vi "FPGA myRIOMain_v7.vi"() -> ()   [LabVIEW 2019]
doc: "Main FPGA VI\nUse the bitfile generated by this VI in the real-time code.\n\nv5: 16-pt Moving Average filter in AI sample loop"
uses:
  <vilib>/eio/EIONode/EIONode.xnode
  <vilib>/rvi/DataTransferAndStorage/Container/XNode/niFpgaContainer.xnode
  <vilib>/rvi/eio/common/nirviEmuTemplateMethod_errors.vi
  <vilib>/rvi/FIFO/Fifo_Resource/nirvififoEmulationRead.vi
  <vilib>/rvi/FIFO/Fifo_Resource/nirvififoEmulationWrite.vi
  FPGA functions/FPGA functions.lvlib
  <vilib>/rvi/FXPMathLib/FxpMul/XNode/nifxpmath_Multiplier.xnode
  <vilib>/rvi/DataTransferAndStorage/Register/Emulation/niFpgaRegisterEmulation.vi
  <vilib>/rvi/Analysis/measure/LMRsmpl/XNode/niFPGA Rational Resampler.xnode
  <vilib>/Platform/TimedLoop/XDataNode/wakeup.ctl
  <vilib>/Platform/TimedLoop/XDataNode/XDNodeRunTimeDep.lvlib
  <vilib>/Platform/TimedLoop/XDataNode/nitl_modes.ctl
  <vilib>/Platform/TimedLoop/XDataNode/timing_clust.ctl
  <vilib>/Platform/TimedLoop/XDataNode/XDataNode.xnode
  <vilib>/rvi/Analysis/common/codeGenErrors/XNode/niFpgaXNodeCodeGenErrorHandle.vi
  <vilib>/rvi/FXPMathLib/sim/FxpSim.dll
  TypeDefs/AO mode TabCtrl.ctl
  TypeDefs/SamplingModeEnum.ctl
panel:
  out "FPGA Proc. \nDMA\nOverflow?":bool
  out "AI M Loop time [ticks]":u32
  out "FPGA AI DMA\nOverflow?":bool
  out "Sample Freq. \ntoo high?":bool
  out "Processing Loop time [ticks]":u32
  in  "Sampling Mode":T1
  in  "AO mode":T2
  in  "AO Out [V]":fxp<+/-,18,5> format="%#.6g"
  in  "AO enable?":bool
  out "AI In [V]":fxp<+/-,24,5> format="%#.6g"
  out "FPGA AO DMA\nOverflow?":bool
  out "Int. Output":i16
  out "Raw Int. Input":fxp<+/-,20,12> format="%.8g"
  out "AO Loop time [ticks]":u32
  out "AI Loop time [ticks]":u32
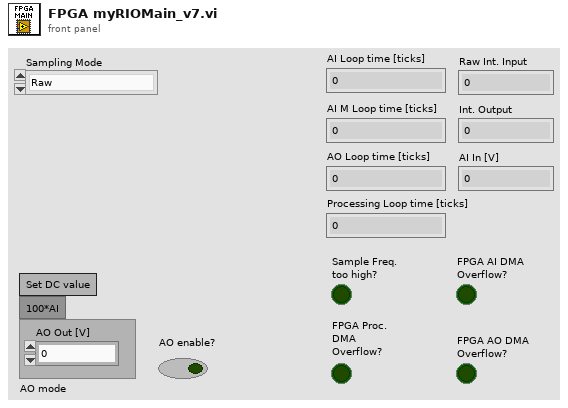
[diagram p1: front panel]
types:
  T1 = typedef "SamplingModeEnum.ctl" = enum16{"Raw", "M64 (ReSpl)", "M128 (ReSpl)", "M256 (ReSpl)", "MA (AI)", "4pt MA (AI) + M64 (ReSpl)", "LPF (Proc.)", "4pt MA (AI) + LPF (Proc.)", "4pt MA (Proc.) + LPF (Proc.)"}
  T2 = typedef "AO mode TabCtrl.ctl" = enum32{"Set DC value", "100*AI"}
  T3 = typedef "XDNodeRunTimeDep.lvlib/timing_clust.ctl" = cluster{"Expected End [f-1]":u64, "Actual End [f-1]":u64, "Finished Late? [f-1]":bool, "Expected End [i-1]":u64, "Actual End [i-1]":u64, "Finished Late? [i-1]":bool, "Expected Start [i]":u64, "Actual Start [i]":u64, "Expected Start [f]":u64, "Actual Start [f]":u64, "Source Name":string, "Structure Name":string, "Period":i64, "Deadline":i64, "Offset":i64, "Start":i64, "Priority":i32, "Timeout":i32, "Mode":T4, "Wakeup Reason":T5, "Error":errorcluster, "Source Type":string, "Secondary Source Type":string, "Global End Time":u64, "Global Start Time":u64, "Frame Duration":u64, "Iteration Duration":u64, "Assigned CPU":i32, "I/O Scan Engine Mode":u32}
  T4 = typedef "XDNodeRunTimeDep.lvlib/nitl_modes.ctl" = enum32{"No Change", "Process missed periods, maintain original phase", "Discard missed periods, maintain original phase", "Process missed periods, ignore original phase", "Discard missed periods, ignore original phase"}
  T5 = typedef "XDNodeRunTimeDep.lvlib/wakeup.ctl" = enum32{"Normal", "Aborted", "Asynchronous wakeup", "Timing source error", "Timed loop error", "Timeout"}
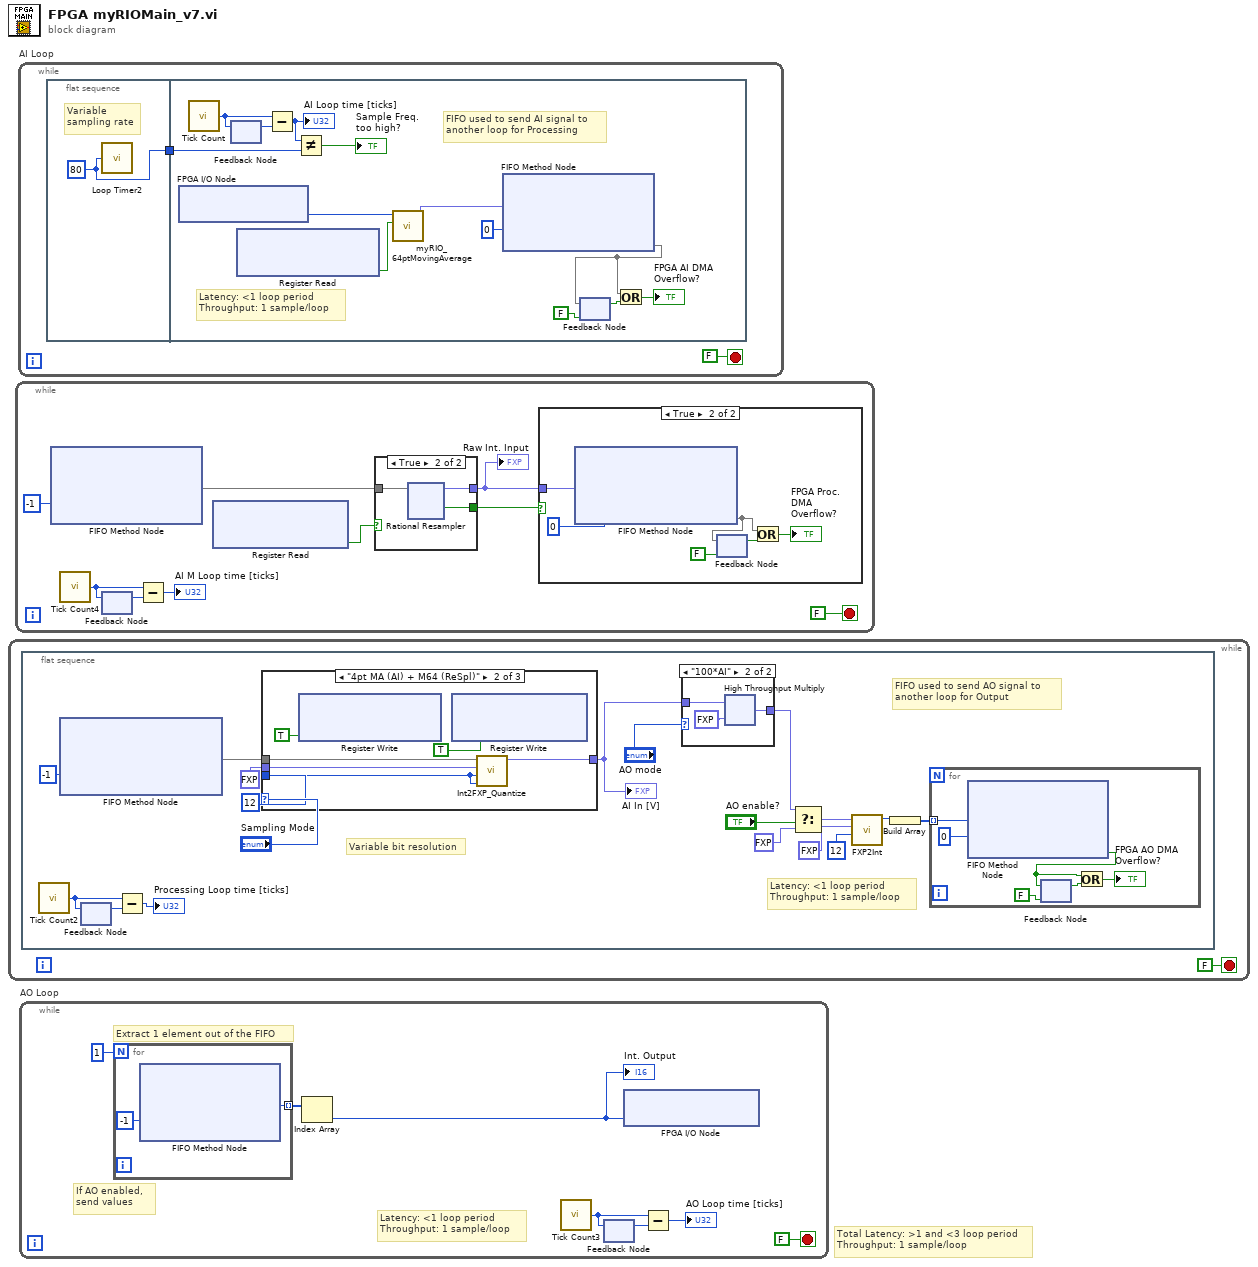
[diagram p0: block diagram]
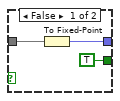
[diagram p3: hidden frame]
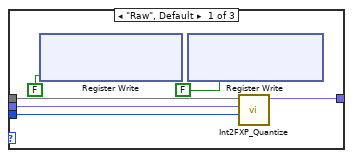
[diagram p4: hidden frame]
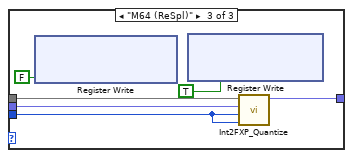
[diagram p5: hidden frame]
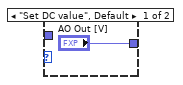
[diagram p6: hidden frame]
diagram:
  # "Total Latency: >1 and <3 loop period\nThroughput: 1 sample/loop"
  n1 = while {
    stop <- FALSE stop-if-true
    n2 = flat-sequence {
      frame #0 {
        # "Variable bit resolution"
        # "Latency: <1 loop period\nThroughput: 1 sample/loop"
        # "FIFO used to send AO signal to \nanother loop for Output"
        n3 = call "Tick Count2"() -> ("Tick Count(Ticks)"=w7:u32)
        n4 = xnode ("FIFO Method Node")("Timeout"=-1) -> ("Element"=w2)  [unwired: 1 in, 2 out]
        n5 = feedback #1() -> (w6:u32)  [unwired: 1 in]
        n6 = feedback-in #1(w7) -> ()
        n7 = Subtract(x=w7, y=w6) -> (x-y=→"Processing Loop time [ticks]":u32)
        n8 = case shown="\"4pt MA (AI) + M64 (ReSpl)\"" "Sampling Mode" {
          tunnel: i8 12 ("Input Bit resolution") -> [w25 w27 w33]
          tunnel: fxp<+,8,4> 10.0 ("Multiplier") -> [w24 w28 w37]
          tunnel: [w23 w30 w36] -> w8
          tunnel: w2 -> [w22 w29 w34]
          frame "Raw", Default {
            n9 = xnode ("Register Write")("Data"=FALSE) -> ()  [unwired: 1 in, 1 out]
            n10 = xnode ("Register Write")("Data"=FALSE) -> ()  [unwired: 1 in, 1 out]
            n11 = call "Int2FXP_Quantize.vi"("Input Bit resolution"=w25, "Multiplier"=w24, "Input (Int)"=w22) -> ("Output (FXP)"=w23:fxp<+/-,24,5>)  [unwired: 8 in]
          }
          frame "4pt MA (AI) + M64 (ReSpl)" {
            n12 = xnode ("Register Write")("Data"=TRUE) -> ()  [unwired: 1 in, 1 out]
            n13 = xnode ("Register Write")("Data"=TRUE) -> ()  [unwired: 1 in, 1 out]
            n14 = call "Int2FXP_Quantize.vi"("Output Bit resolution"=w27, "Input Bit resolution"=w27, "Multiplier"=w28, "Input (Int)"=w29) -> ("Output (FXP)"=w30:fxp<+/-,24,5>)  [unwired: 7 in]
          }
          frame "M64 (ReSpl)" {
            n15 = xnode ("Register Write")("Data"=FALSE) -> ()  [unwired: 1 in, 1 out]
            n16 = xnode ("Register Write")("Data"=TRUE) -> ()  [unwired: 1 in, 1 out]
            n17 = call "Int2FXP_Quantize.vi"("Output Bit resolution"=w33, "Input Bit resolution"=w33, "Multiplier"=w37, "Input (Int)"=w34) -> ("Output (FXP)"=w36:fxp<+/-,24,5>)  [unwired: 7 in]
          }
        }
        "AI In [V]" <- w8
        n18 = case shown="\"100*AI\"" "AO mode" {
          tunnel: ["AO Out [V]" w39] -> w12
          tunnel: w8 -> [_ w41]
          frame "Set DC value", Default {
          }
          frame "100*AI" {
            n19 = xnode ("High Throughput Multiply")("x"=w41, "y"=fxp<+,5,7> 100.0) -> ("x*y"=w39:fxp<+/-,18,5>)
          }
        }
        n20 = Select(t=w12, s="AO enable?", f=fxp<+/-,18,5> 0.0) -> (s? t:f=w13:fxp<+/-,18,5>)
        n21 = call "FXP2Int.vi"("Output Bit resolution"=i8 12 ("Bit resolution"), "Multiplier"=fxp<+,18,-1> 0.10000038146972656, "Input (FXP)"=w13) -> ("Output (Int)"=w19:i16)  [unwired: 8 in]
        n22 = Build Array(w19) -> (w14:i16[])
        n23 = for {
          tunnel: w14 -> [w44] mode=indexing
          n24 = xnode ("FIFO Method Node")("Element"=w44, "Timeout"=0) -> ("Timed Out?"=w42:bool)  [unwired: 1 in, 1 out]
          n25 = feedback-in #2(w42) -> ()
          n26 = feedback #2(FALSE ("Timed Out?")) -> (w46:bool)
          n27 = Or(x=w42, y=w46) -> (x .or. y?=→"FPGA AO DMA\nOverflow?":bool)
        }
      }
    }
  }
  n28 = while {
    stop <- FALSE stop-if-true
    n29 = xnode ("FIFO Method Node")("Timeout"=-1) -> ("Element"=w51)  [unwired: 1 in, 2 out]
    n30 = call "Tick Count4"() -> ("Tick Count(Ticks)"=w55:u32)
    n31 = feedback #3() -> (w54:u32)  [unwired: 1 in]
    n32 = feedback-in #3(w55) -> ()
    n33 = Subtract(x=w55, y=w54) -> (x-y=→"AI M Loop time [ticks]":u32)
    n34 = xnode ("Register Read")() -> ("Data"=w50:bool)  [unwired: 1 in, 1 out]
    n35 = case shown="True" w50 {
      tunnel: w51 -> [w64 w68]
      tunnel: [w65 w67] -> w48
      tunnel: [TRUE ("output valid") w66] -> w49
      frame False {
        n36 = To Fixed-Point(number=w64) -> (fixed-point=w65:fxp<+/-,18,12>)  [unwired: 1 in]
      }
      frame True {
        n37 = xnode "Rational Resampler"("input data"=w68) -> ("output data"=w67:fxp<+/-,20,12>, "output valid"=w66:bool)  [unwired: 1 out]
      }
    }
    "Raw Int. Input" <- w48
    n38 = case shown="True" w49 {
      tunnel: w48 -> [_ w61]
      frame False {
      }
      frame True {
        n39 = xnode ("FIFO Method Node")("Element"=w61, "Timeout"=0) -> ("Timed Out?"=w57)  [unwired: 1 in, 1 out]
        n40 = feedback #4(FALSE ("Timed Out?")) -> (w59:bool)
        n41 = feedback-in #4(w57) -> ()
        n42 = Or(x=w57, y=w59) -> (x .or. y?=→"FPGA Proc. \nDMA\nOverflow?":bool)
      }
    }
  }
  n43 = while "AI Loop" {
    stop <- FALSE stop-if-true
    n44 = flat-sequence {
      tunnel: [w105] -> w103
      tunnel: w103 -> [w115]
      frame #0 {
        w105 = u32 80 ("Sample Time [ticks]")
        # "Variable\nsampling rate"
        n45 = call "Loop Timer2"("Count(Ticks)"=w105) -> ()  [unwired: 1 out]
      }
      frame #1 {
        # "FIFO used to send AI signal to \nanother loop for Processing"
        # "Latency: <1 loop period\nThroughput: 1 sample/loop"
        n46 = xnode "FPGA I/O Node"() -> ("ConnectorC/AI0"=w108:i16)  [unwired: 1 in, 1 out]
        n47 = call "Tick Count"() -> ("Tick Count(Ticks)"=w118:u32)
        n48 = feedback #5() -> (w117:u32)  [unwired: 1 in]
        n49 = feedback-in #5(w118) -> ()
        n50 = xnode ("Register Read")() -> ("Data"=w106:bool)  [unwired: 1 in, 1 out]
        n51 = Subtract(x=w118, y=w117) -> (x-y=w116:u32)
        "AI Loop time [ticks]" <- w116
        n52 = Not Equal?(x=w116, y=w115) -> (x != y?=→"Sample Freq. \ntoo high?":bool)
        n53 = call "myRIO_64ptMovingAverage.vi"("Enable?"=w106, "Raw input"=w108) -> ("Avg. output"=w107:fxp<+/-,18,12>)  [unwired: 9 in]
        n54 = xnode ("FIFO Method Node")("Element"=w107, "Timeout"=0) -> ("Timed Out?"=w109)  [unwired: 1 in, 1 out]
        n55 = feedback #6(FALSE ("Timed Out?")) -> (w111:bool)
        n56 = feedback-in #6(w109) -> ()
        n57 = Or(x=w109, y=w111) -> (x .or. y?=→"FPGA AI DMA\nOverflow?":bool)
      }
    }
  }
  n58 = while "AO Loop" {
    stop <- FALSE stop-if-true
    # "Latency: <1 loop period\nThroughput: 1 sample/loop"
    # "If AO enabled, \nsend values"
    # "Extract 1 element out of the FIFO"
    n59 = for {
      N: 1 -> [_]
      tunnel: [w127] -> w121 mode=indexing
      n60 = xnode ("FIFO Method Node")("Timeout"=-1) -> ("Element"=w127:i16)  [unwired: 1 in, 2 out]
    }
    n61 = Index Array(array=w121) -> (element=w119:i16)  [unwired: 1 in]
    "Int. Output" <- w119
    n62 = call "Tick Count3"() -> ("Tick Count(Ticks)"=w124:u32)
    n63 = feedback #7() -> (w123:u32)  [unwired: 1 in]
    n64 = feedback-in #7(w124) -> ()
    n65 = xnode "FPGA I/O Node"("ConnectorC/AO0"=w119) -> ()  [unwired: 1 in, 1 out]
    n66 = Subtract(x=w124, y=w123) -> (x-y=→"AO Loop time [ticks]":u32)
  }
